vi "WSVCAP SHL FPGA LL Configuration File Handler.vi"(0 "Object Cluster In":T3={"Settings"={"I2C Slave Address"=144, "I2C Clock Rate (Hz)"=20.0, "SPI Clock Rate (Hz)"=50000.0, "RFFE Slave Address"=255, "RFFE Clock Rate (Hz)"=20.0, "Simulate FPGA"=TRUE, "C1 Cap DAC Default"=165, "C2 Cap DAC Default"=165, "C3 Cap DAC Default"=134, "C4 Cap DAC Default"=150}, "FPGA Resource"="", "Online"=FALSE, "I2C Wait Ticks"=0, "SPI Wait Ticks"=0, "RFFE Wait Ticks"=0, "FPGA VI Reference (FPGA Mode)"=refnum, "FPGA VI Reference (Sim Mode)"=refnum} {"Settings"."C4 Cap DAC Default" format="0x%02x"; "Settings"."C3 Cap DAC Default" format="0x%02x"; "Settings"."C2 Cap DAC Default" format="0x%02x"; "Settings"."C1 Cap DAC Default" format="0x%02x"; "Settings"."RFFE Clock Rate (Hz)" format="%.0f Hz"; "Settings"."RFFE Slave Address" format="0x%02x"; "Settings"."I2C Clock Rate (Hz)" format="%.0f Hz"; "Settings"."SPI Clock Rate (Hz)" format="%.0f Hz"; "Settings"."I2C Slave Address" format="0x%02x"}, 1 "Copy Path":path, 2 "System Cfg":T2={"Configuration File Path"=path "inifiles/System Configuration.ini"}, 7 "Copy Tag":string, 11 "Error In (no error)":errorcluster, 12 "Keys (Empty:All)":T1[](array[typedef]), 13 "Operation":T6) -> (4 "Object Cluster Out":T3={"Settings"={"I2C Slave Address"=144, "I2C Clock Rate (Hz)"=20.0, "SPI Clock Rate (Hz)"=50000.0, "RFFE Slave Address"=255, "RFFE Clock Rate (Hz)"=20.0, "Simulate FPGA"=TRUE, "C1 Cap DAC Default"=165, "C2 Cap DAC Default"=165, "C3 Cap DAC Default"=134, "C4 Cap DAC Default"=150}, "FPGA Resource"="", "Online"=FALSE, "I2C Wait Ticks"=0, "SPI Wait Ticks"=0, "RFFE Wait Ticks"=0, "FPGA VI Reference (FPGA Mode)"=refnum, "FPGA VI Reference (Sim Mode)"=refnum} {"Settings"."C4 Cap DAC Default" format="0x%02x"; "Settings"."C3 Cap DAC Default" format="0x%02x"; "Settings"."C2 Cap DAC Default" format="0x%02x"; "Settings"."C1 Cap DAC Default" format="0x%02x"; "Settings"."RFFE Clock Rate (Hz)" format="%.0f Hz"; "Settings"."RFFE Slave Address" format="0x%02x"; "Settings"."I2C Clock Rate (Hz)" format="%.0f Hz"; "Settings"."SPI Clock Rate (Hz)" format="%.0f Hz"; "Settings"."I2C Slave Address" format="0x%02x"}, 8 "Cancelled":bool, 15 "Error Out":errorcluster)   [LabVIEW 2017]
uses:
  Type Defs/WSVCAP SHL Core System Cluster.ctl
  Type Defs/WSVCAP SHL I2C Settings Cluster.ctl
  Type Defs/WSVCAP SHL FPGA Ref.ctl
  user.lib/Configuration Files/Type Defs/CFG File Operation Enum.ctl
  Type Defs/WSVCAP SHL Configuration Items Enum.ctl
  user.lib/Configuration Files/Type Defs/CFG System Configuration Settings Cluster.ctl
panel:
  in  "Config Enum":T1=enum."Settings::Simulate FPGA"
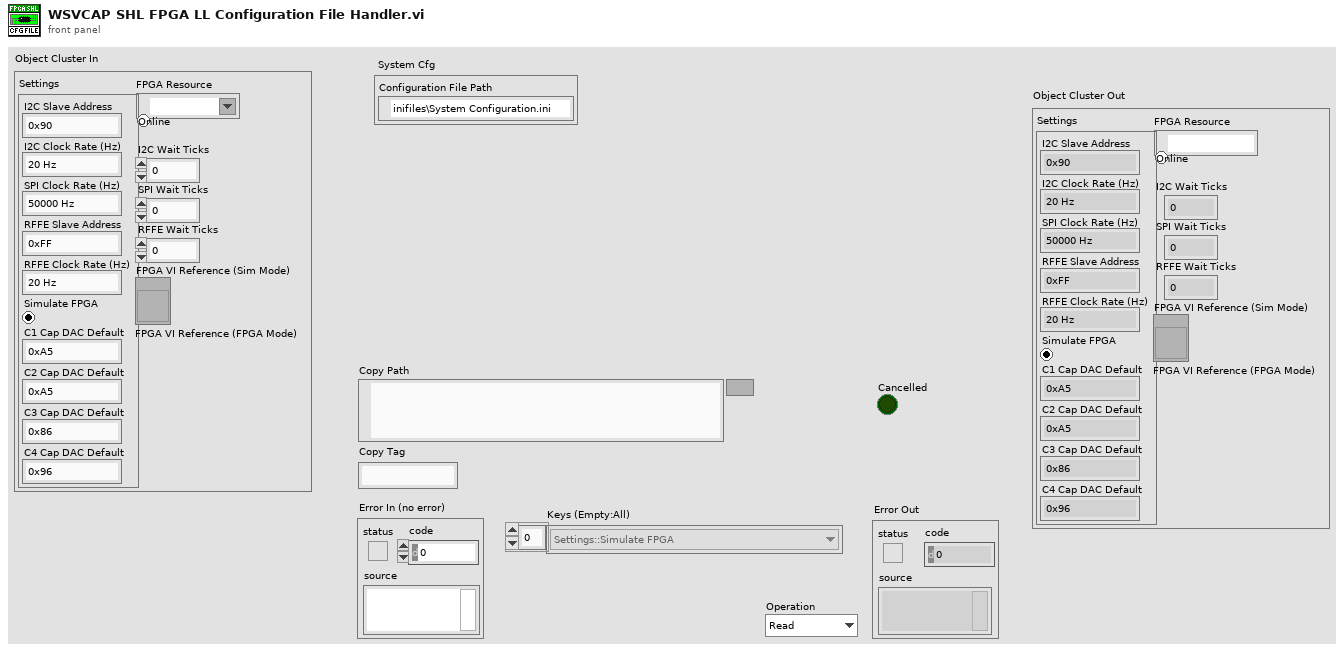
[diagram p1: front panel]
types:
  T1 = typedef "WSVCAP SHL Configuration Items Enum.ctl" = enum16{"Settings::I2C Slave Address", "Settings::I2C Clock Rate (Hz)", "Settings::C1 Cap DAC Default", "Settings::C2 Cap DAC Default", "Settings::C3 Cap DAC Default", "Settings::C4 Cap DAC Default", "Settings::SPI Clock Rate (Hz)", "Settings::RFFE Slave Address", "Settings::RFFE Clock Rate (Hz)", "Settings::Simulate FPGA"}
  T2 = typedef "CFG System Configuration Settings Cluster.ctl" = cluster{"Configuration File Path":path}
  T3 = typedef "WSVCAP SHL Core System Cluster.ctl" = cluster{"Settings":T4, "FPGA Resource":tag, "Online":bool, "I2C Wait Ticks":u32, "SPI Wait Ticks":u32, "RFFE Wait Ticks":u32, "FPGA VI Reference (FPGA Mode)":T5, "FPGA VI Reference (Sim Mode)":refnum<vi>}
  T4 = typedef "WSVCAP SHL I2C Settings Cluster.ctl" = cluster{"I2C Slave Address":u8, "I2C Clock Rate (Hz)":dbl, "SPI Clock Rate (Hz)":dbl, "RFFE Slave Address":u8, "RFFE Clock Rate (Hz)":dbl, "Simulate FPGA":bool, "C1 Cap DAC Default":u8, "C2 Cap DAC Default":u8, "C3 Cap DAC Default":u8, "C4 Cap DAC Default":u8}
  T5 = typedef "WSVCAP SHL FPGA Ref.ctl" = refnum<k20>
  T6 = typedef "CFG File Operation Enum.ctl" = enum16{"Read", "Write", "Copy", "Edit"}
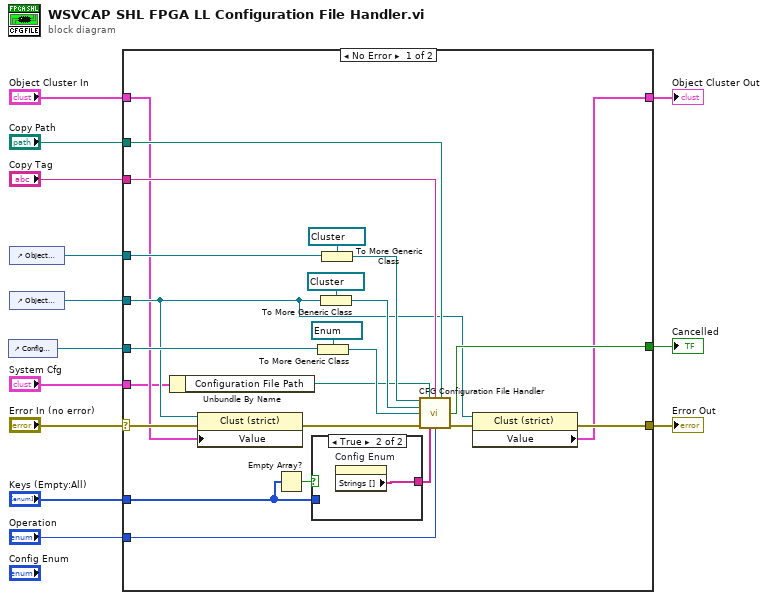
[diagram p0: block diagram]
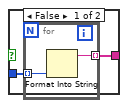
[diagram p2: hidden frame]
diagram:
  n1 = control-ref of="Config Enum"() -> (w2:refnum<vi>)
  n2 = control-ref of="Object Cluster In"() -> (w3:refnum<vi>)
  n3 = control-ref of="Object Cluster Out"() -> (w1:refnum<vi>)
  n4 = case shown="No Error" "Error In (no error)" {
    selector: "Error In (no error)" -> [w20 w44]
    tunnel: [w33 w44] -> w11
    tunnel: "Copy Path" -> [w35 _]
    tunnel: "Copy Tag" -> [w36 _]
    tunnel: "Operation" -> [w37 _]
    tunnel: [w14 w43] -> w7
    tunnel: "Object Cluster In" -> [w17 w43]
    tunnel: w3 -> [w29 _]
    tunnel: w1 -> [w18 _]
    tunnel: w2 -> [w28 _]
    tunnel: "Keys (Empty:All)" -> [w24 _]
    tunnel: [w21 _] -> w5
    tunnel: "System Cfg" -> [w16 _]
    frame No Error {
      n5 = Unbundle By Name(w16) -> ("Configuration File Path"=w15:path)
      n6 = property class="Clust (strict)"(reference=w18, error in=w20, "Value"=w17) -> (error out=w19:errorcluster)  [unwired: 1 out]
      n7 = Empty Array?(array=w24) -> (empty?=w23:bool)
      n8 = case shown="True" w23 {
        tunnel: w24 -> [w39 _]
        tunnel: [w38 w42] -> w22
        frame False {
          n9 = for {
            tunnel: w39 -> [w41] mode=indexing
            tunnel: [w40] -> w38 mode=indexing
            n10 = Format Into String(w41) -> (resulting string=w40:string)  [unwired: 3 in, 1 out]
          }
        }
        frame True {
          n11 = property on="Config Enum" class="Enum (strict)"() -> ("Strings []"=w42:string[])  [unwired: 2 in, 2 out]
        }
      }
      n12 = To More Generic Class(target class=refnum<vi> refnum ("Enum Ref"), reference=w28) -> (generic class reference=w25:refnum<vi>)
      n13 = To More Generic Class(target class=refnum<vi> refnum ("Cluster Ref"), reference=w18) -> (generic class reference=w26:refnum<vi>)
      n14 = To More Generic Class(target class=refnum<vi> refnum ("Cluster Ref"), reference=w29) -> (generic class reference=w27:refnum<vi>)
      n15 = call "CFG Configuration File Handler.vi"("Cluster In Ref"=w27, "System Configuration File"=w15, "Copy Tag"=w36, "Copy Path"=w35, "Cluster Out Ref"=w26, "Enum Ref"=w25, "Error In (no error)"=w19, "Keys (Empty:All)"=w22, "Operation"=w37) -> ("Cancelled"=w21:bool, "Error Out"=w34:errorcluster)  [unwired: 5 in]
      n16 = property class="Clust (strict)"(reference=w18, error in=w34) -> (error out=w33:errorcluster, "Value"=w14:T3)  [unwired: 1 out]
    }
    frame Error {
    }
  }
  "Object Cluster Out" <- w7
  "Error Out" <- w11
  "Cancelled" <- w5
